vi "FunctDataMgr.Function Return.vi"(6 "RTN Info":variant, 8 "Error In":errorcluster, 10 "RTN Vars":variant, 11 "FunctDataMgr in":refnum<class "FunctDataMgr.lvclass">) -> (0 "Error Out":errorcluster, 3 "FunctDataMgr out":refnum<class "FunctDataMgr.lvclass">)   [LabVIEW 2018, in "FunctDataMgr.lvclass"]
uses:
  FunctDataMgr.lvclass
  <vilib>/KATE/Queues/Q.Msg Return Data Container.ctl
  FunctDataMgr.lvclass/FunctDataMgr.ctl
  TestExec/TestExec.Local Result Data.ctl
  Results/Result.Attribute.ctl
  Results/Result.Measurement and Attribute Item Status.ctl
  Results/Result.Numeric.ctl
  Results/Result.Limit Type.ctl
  Results/Result XML/TestResult.SW Item.ctl
  Reports/Report.Result FileDataObject.ctl
  Results/Result.Measurement Item.ctl
  <vilib>/KATE/Queues/Queue Utils.lvlib
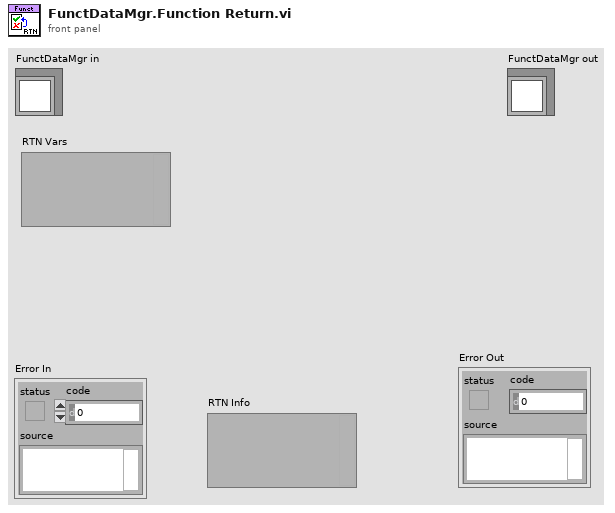
[diagram p1: front panel]
types:
  T1 = typedef "KATE_Lib.lvlib/Queue Utils.lvlib/Q.Msg Return Data Container.ctl" = cluster{"SeqNum":i32, "Data":variant, "Error":errorcluster}
  T2 = typedef "TestExec.Local Result Data.ctl" = cluster{"Attr":T3[], "Num":T5[], "UUT Props":string[][], "Vars":string[][], "SW Items":T7[], "Error":errorcluster, "Step":i32, "FileObjs":T8[], "MeasData":T9[]}
  T3 = typedef "Result.Attribute.ctl" = cluster{"Cnt":i32, "Step":string, "Category":string, "Name":string, "Value":string, "Status":T4, "Code":i32, "Desc":string, "Time":timestamp}
  T4 = typedef "Result.Measurement and Attribute Item Status.ctl" = i32
  T5 = typedef "Result.Numeric.ctl" = cluster{"Cnt":i32, "Step":string, "Category":string, "Name":string, "Value":dbl, "Units":string, "LimType":T6, "LL":dbl, "UL":dbl, "Status":T4, "Code":i32, "Desc":string, "Time":timestamp}
  T6 = typedef "Result.Limit Type.ctl" = enum16{"None", "EQ", "NE", "GT", "LT", "GE", "LE", "GTLT", "GELE", "GELT", "GTLE", "LTGT", "LEGE", "LEGT", "LTGE", "Contains", "NotContains"}
  T7 = typedef "TestResult.SW Item.ctl" = cluster{"Name":string, "PN":string, "Version":string, "Note":string}
  T8 = typedef "Report.Result FileDataObject.ctl" = cluster{"Cnt":i32, "Step":string, "Category":string, "Name":string, "Type":string, "File Name":string, "Time":string, "Path":path}
  T9 = typedef "Result.Measurement Item.ctl" = cluster{"Cnt":i32, "Step":string, "Category":string, "Name":string, "Value":string, "Units":string, "LimType":string, "LL":string, "UL":string, "Status":T4, "Code":i32, "Desc":string, "Time":timestamp}
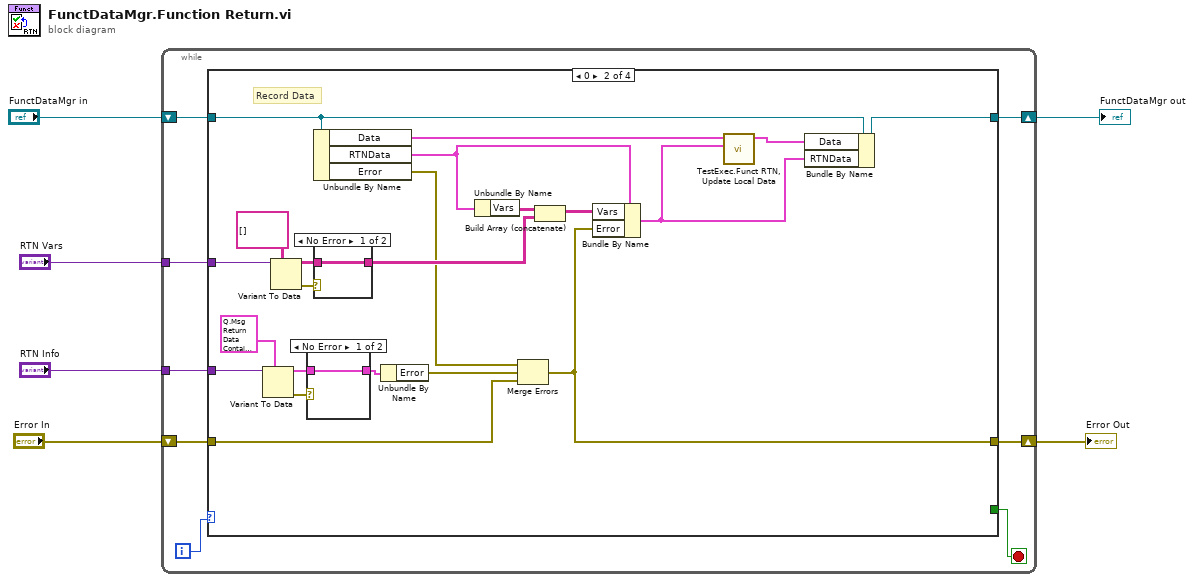
[diagram p0: block diagram]
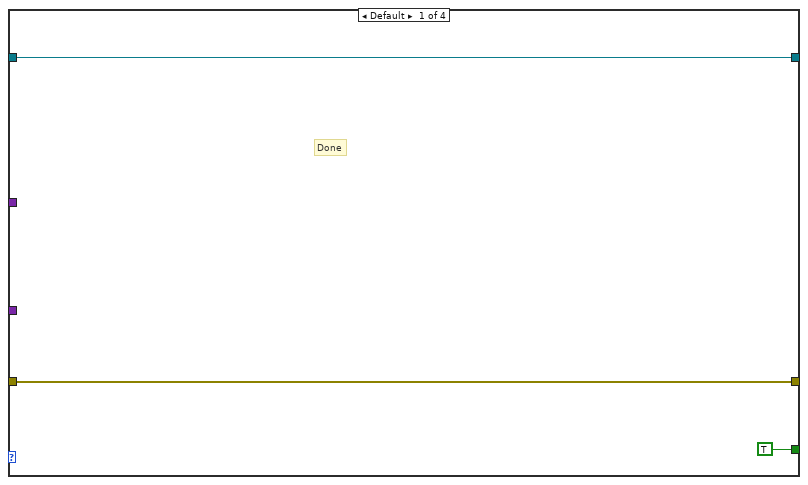
[diagram p2: hidden frame]
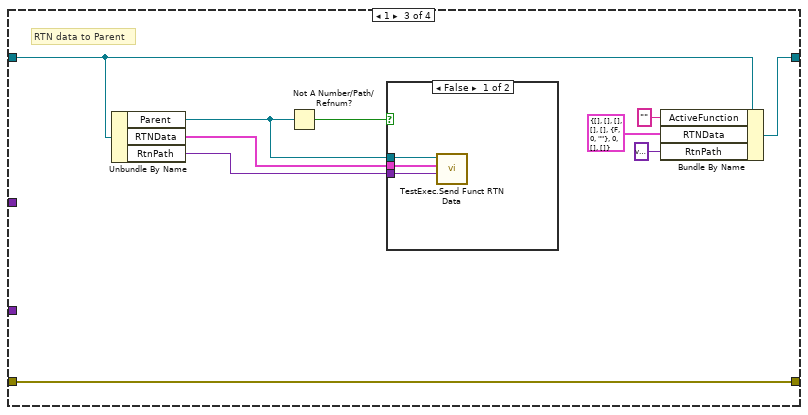
[diagram p5: hidden frame]
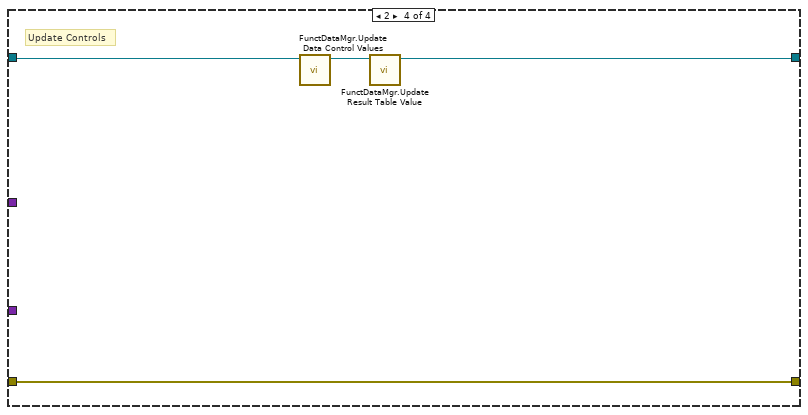
[diagram p7: hidden frame]
diagram:
  n1 = while {
    tunnel: "RTN Vars" -> [w14]
    tunnel: "RTN Info" -> [w13]
    shift-right: [w11] -> w5
    shift-left: "FunctDataMgr in" -> [w12]
    shift-right: [w7] -> w1
    shift-left: "Error In" -> [w10]
    i -> [w9]
    stop <- w8 stop-if-true
    n2 = case shown="0" w9 {
      tunnel: w14 -> [_ w35 _ _]
      tunnel: w13 -> [_ w34 _ _]
      tunnel: w12 -> [w17 w28 w47 w57]
      tunnel: [w17 w26 w46 w55] -> w11
      tunnel: w10 -> [w15 w20 w42 w58]
      tunnel: [TRUE _ _ _] -> w8
      tunnel: [w15 w19 w42 w58] -> w7
      frame Default {
        # "Done"
      }
      frame 0 {
        # "Record Data"
        n3 = Variant To Data(type=T1 {"SeqNum"=0, "Data"=variant, "Error"={"status"=FALSE, "code"=0, "source"=""}} ("Ret"), Variant=w34) -> (data=w23:T1, error out=w24:errorcluster)  [unwired: 1 in]
        n4 = Variant To Data(type=string[][] [], Variant=w35) -> (data=w37:string[][], error out=w38:errorcluster)  [unwired: 1 in]
        n5 = case shown="No Error" w24 {
          tunnel: w23 -> [w40 _]
          tunnel: [w40 _] -> w22
          frame No Error {
          }
          frame Error {
          }
        }
        n6 = Unbundle By Name(w28) -> ("Data"=w29:T2, "RTNData"=w30:T2, "Error"=w18:errorcluster)
        n7 = case shown="No Error" w38 {
          tunnel: w37 -> [w41 _]
          tunnel: [w41 _] -> w31
          frame No Error {
          }
          frame Error {
          }
        }
        n8 = Unbundle By Name(w22) -> ("Error"=w21:errorcluster)
        n9 = Unbundle By Name(w30) -> ("Vars"=w33:string[][])
        n10 = Merge Errors(w18, w21, w20) -> (w19:errorcluster)
        n11 = Build Array (concatenate)(w33, w31) -> (w32:string[][])
        n12 = Bundle By Name(cluster=w30, "Vars"=w32, "Error"=w19) -> (w25:T2)
        n13 = call "TestExec.Funct RTN, Update Local Data.vi"("RTN Data"=w25, "Local Data"=w29) -> ("Local Data Out"=w27:T2)  [unwired: 9 in]
        n14 = Bundle By Name(cluster=w28, "Data"=w27, "RTNData"=w25) -> (w26:refnum<class "FunctDataMgr.lvclass">)
      }
      frame 1 {
        # "RTN data to Parent"
        n15 = Unbundle By Name(w47) -> ("Parent"=w49:refnum<queue>, "RTNData"=w51:T2, "RtnPath"=w50:variant)
        n16 = Not A Number/Path/Refnum?(number/path/refnum=w49) -> (NaN/Path/Refnum?=w48:bool)
        n17 = case shown="False" w48 {
          tunnel: w51 -> [w54 _]
          tunnel: w50 -> [w53 _]
          tunnel: w49 -> [w52 _]
          frame False {
            n18 = call "TestExec.Send Funct RTN Data.vi"("RTN Route (Data2)"=w53, "RTN Data"=w54, "Q In"=w52) -> ()  [unwired: 8 in, 1 out]
          }
          frame True {
          }
        }
        n19 = Bundle By Name(cluster=w47, "ActiveFunction"="", "RTNData"=T2 {"Attr"=[], "Num"=[], "UUT Props"=[], "Vars"=[], "SW Items"=[], "Error"={"status"=FALSE, "code"=0, "source"=""}, "Step"=0, "FileObjs"=[], "MeasData"=[]}, "RtnPath"=variant) -> (w46:refnum<class "FunctDataMgr.lvclass">)
      }
      frame 2 {
        # "Update Controls"
        n20 = call "FunctDataMgr.Update Data Control Values.vi"("FunctDataMgr in"=w57) -> ("FunctDataMgr out"=w56:refnum<class "FunctDataMgr.lvclass">)  [unwired: 9 in, 1 out]
        n21 = call "FunctDataMgr.Update Result Table Value.vi"("FunctDataMgr in"=w56) -> ("FunctDataMgr out"=w55:refnum<class "FunctDataMgr.lvclass">)  [unwired: 9 in, 1 out]
      }
    }
  }
  "FunctDataMgr out" <- w5
  "Error Out" <- w1
